vi "Drop Message Core.vi"(11 "Flush Sequncer Msg in":refnum<class "Flush Sequncer Msg.lvclass">) -> ()   [LabVIEW 2020, in "Sequencer.lvlib" / "Flush Sequncer Msg.lvclass"]
doc: "(<B>Filename</B>: Actor Framework.lvlib:Message.lvclass:Drop Message Core.vi)\n\nDefines what a message does if it is in the message queue when the queue is released. At this point, the actor has shut down, so it will never process the message.\n\nRelease the status notifier preventing a stall on the Sequencer."
uses:
  Flush Sequncer Msg.lvclass
  Flush Sequncer Msg.lvclass/Flush Sequncer Msg.ctl
  PPL/HDH.Data.Generic.lvlibp/Synchronization/Notifier/Notifier.lvclass
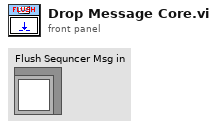
[diagram p1: front panel]
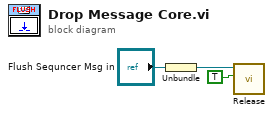
[diagram p0: block diagram]
diagram:
  n1 = Unbundle("Flush Sequncer Msg in") -> (w1:refnum<class "Notifier.lvclass">)
  n2 = call "Release.vi"("Force destroy? (F)"=TRUE, "Notifier in"=w1) -> ()  [unwired: 7 in, 3 out]
